vi "m1m3shmmonitorCommandMoveHardpointActuators.vi"(8 "error in (no error)":errorcluster, 11 "command_MoveHardpointActuators_Ctl":T1={"Steps[6]"=[0, 0, 0, 0, 0, 0]}) -> (0 "error out":errorcluster, 2 "function return":i32, 3 "command_MoveHardpointActuators_Ctl out":T1)   [LabVIEW 2016, in "SALLV_m1m3.lvlib"]
doc: "int m1m3_shm_monitorCommand_MoveHardpointActuatorsLV(m1m3_command_MoveHardpointActuatorsLV *command_MoveHardpointActuators_Ctl );"
uses:
  SALLV_m1m3.lvlib
  DataTypes/command_MoveHardpointActuators.ctl
  SALLV_m1m3.so
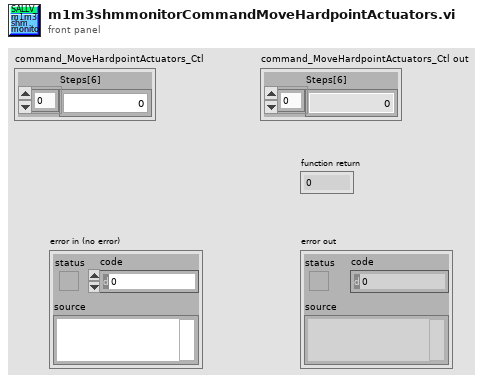
[diagram p1: front panel]
types:
  T1 = typedef "SALLV_m1m3.lvlib/command_MoveHardpointActuators.ctl" = cluster{"Steps[6]":i32[]}
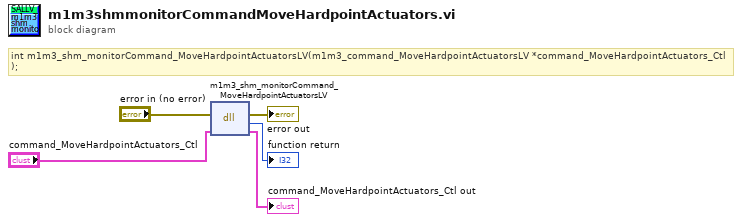
[diagram p0: block diagram]
diagram:
  # "int m1m3_shm_monitorCommand_MoveHardpointActuatorsLV(m1m3_command_MoveHardpointActuatorsLV *command_MoveHardpointActuators_Ctl );"
  n1 = dll-call lib="opt/CODE/SALLV_m1m3/SALLV_m1m3.*" fn="m1m3_shm_monitorCommand_MoveHardpointActuatorsLV"(error in="error in (no error)", "command_MoveHardpointActuators_Ctl"="command_MoveHardpointActuators_Ctl") -> (error out=→"error out":errorcluster, →"function return":i32, "command_MoveHardpointActuators_Ctl"=→"command_MoveHardpointActuators_Ctl out":T1)  [unwired: 2 in, 1 out]
